vi "prepareStiffnessBaseline.vi"(8 "error in (no error)":errorcluster, 11 "Model in":refnum<class "Model.lvclass">) -> (0 "error out":errorcluster, 3 "Model out":refnum<class "Model.lvclass">)   [LabVIEW 2013]
uses:
  ApplicationElements/StiffnessMonitor/StiffnessMonitor.lvclass
  <userlib>/Common/Devices/ForceSensorCalculator/ForceSensorCalculator/ForceSensorCalculator.lvclass
  <userlib>/Common/Devices/EncoderConverter/EncoderConverter/EncoderConverter.lvclass
  <userlib>/Common/Devices/DistanceGauge/DistanceGauge/DistanceGauge.lvclass
  Model.lvclass
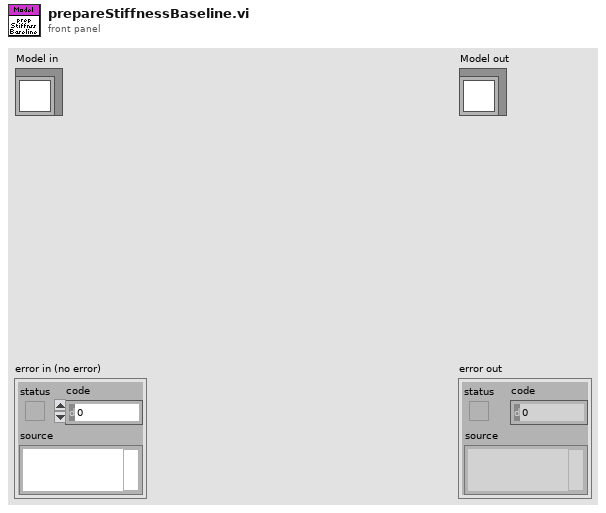
[diagram p1: front panel]
types:
  T1 = typedef "DistanceGauge.lvlib/Distance Data.ctl" = cluster{"Distance Measured 1":dbl[unit], "Distance Measured 2":dbl[unit]}
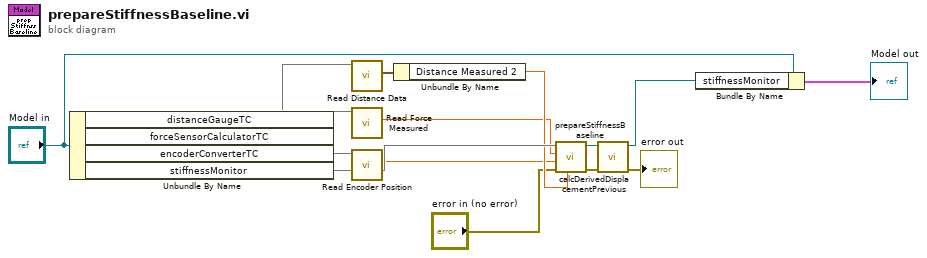
[diagram p0: block diagram]
diagram:
  n1 = Unbundle By Name("Model in") -> ("distanceGaugeTC"=w5, "forceSensorCalculatorTC"=w12, "encoderConverterTC"=w10, "stiffnessMonitor"=w15)
  n2 = call <userlib>:"Read Distance Data.vi"("DistanceGauge in"=w5) -> ("Distance Data"=w4:T1)  [unwired: 9 in, 1 out]
  n3 = call <userlib>:"Read Force Measured.vi"("ForceSensor in"=w12) -> ("Force Demand"=w11:dbl[unit])  [unwired: 9 in, 1 out]
  n4 = call <userlib>:"Read Encoder Position.vi"("EnccoderConverter in"=w10) -> ("EnccoderConverter Position"=w9:dbl[unit])  [unwired: 9 in, 1 out]
  n5 = Unbundle By Name(w4) -> ("Distance Measured 2"=w13:dbl[unit])
  n6 = call "prepareStiffnessBaseline.vi"("Distance to Plate Measured"=w13, "error in (no error)"="error in (no error)", "Encoder Position"=w9, "Force Measured"=w11, "StiffnessMonitor in"=w15) -> ("error out"=w2:errorcluster, "StiffnessMonitor out"=w14:refnum<class "StiffnessMonitor.lvclass">)  [unwired: 5 in]
  n7 = call "calcDerivedDisplacementPrevious.vi"("error in (no error)"=w2, "StiffnessMonitor in"=w14) -> ("error out"=→"error out":errorcluster, "StiffnessMonitor out"=w8:refnum<class "StiffnessMonitor.lvclass">)  [unwired: 8 in]
  n8 = Bundle By Name(cluster="Model in", "stiffnessMonitor"=w8) -> (→"Model out":cluster{})
